vi "Validación Experimental.vi"() -> ()   [LabVIEW 2013]
uses:
  <vilib>/Instr/_visa.llb/VISA Configure Serial Port (Instr).vi
panel:
  in  "Tiempo en alto [us]":i64(knob) scale=1000.0..2000.0
  out "Datos enviados":string
  in  "stop":bool
  in  "Puerto Serial":refnum<visa-resource-name>
  # "Validación Experimental del Modelo"
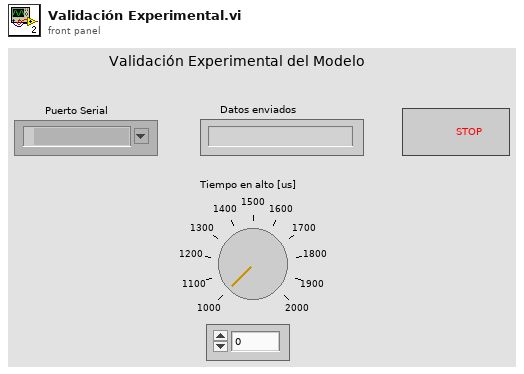
[diagram p1: front panel]
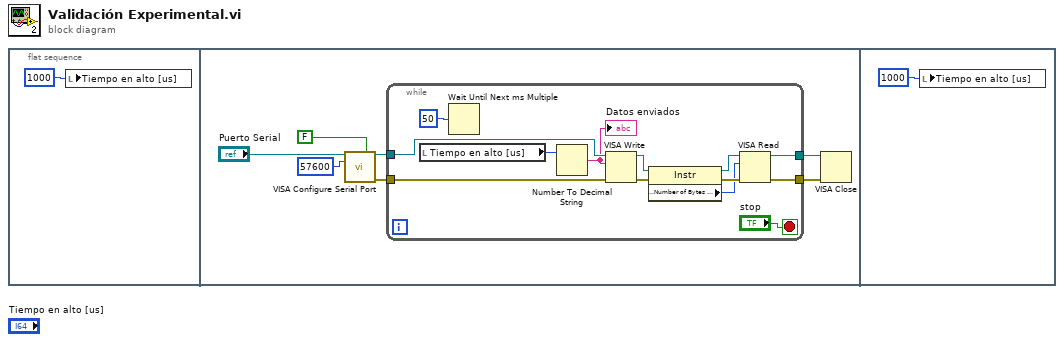
[diagram p0: block diagram]
diagram:
  n1 = flat-sequence {
    frame #0 {
      n2 = local write "Tiempo en alto [us]"(i64 1000 ("Dial")) -> ()
    }
    frame #1 {
      n3 = call-poly "VISA Configure Serial Port"("VISA resource name"="Puerto Serial", "Enable Termination\nChar (T)"=FALSE ("Enable Termination\nChar (T)"), "baud rate (9600)"=u32 57600) -> ("VISA resource name out"=w7:refnum<visa-resource-name>, "error out"=w5:errorcluster)  [unwired: 11 in]
      n4 = while {
        tunnel: w7 -> [w18]
        tunnel: [w16] -> w6
        tunnel: w5 -> [w15]
        tunnel: [w13] -> w4
        stop <- "stop" stop-if-true
        n5 = local read "Tiempo en alto [us]"() -> (w10:i64)
        n6 = Wait Until Next ms Multiple(millisecond multiple=u32 50) -> ()  [unwired: 1 out]
        n7 = Number To Decimal String(number=w10) -> (decimal integer string=w9:string)  [unwired: 1 in]
        "Datos enviados" <- w9
        n8 = VISA Write(VISA resource name=w18, write buffer=w9, error in (no error)=w15) -> (VISA resource name out=w17:refnum<visa-resource-name>, error out=w14:errorcluster)  [unwired: 1 out]
        n9 = property class="Instr"(reference=w17, error in=w14) -> (reference out=w19:refnum<visa-resource-name>, error out=w21:errorcluster, "Serial Settings:Number of Bytes at Serial Port"=w20:u32)
        n10 = VISA Read(VISA resource name=w19, byte count=w20, error in (no error)=w21) -> (VISA resource name out=w16:refnum<visa-resource-name>, error out=w13:errorcluster)  [unwired: 2 out]
      }
      n11 = VISA Close(VISA resource name=w6, error in (no error)=w4) -> ()  [unwired: 1 out]
    }
    frame #2 {
      n12 = local write "Tiempo en alto [us]"(i64 1000 ("Dial")) -> ()
    }
  }
